vi "单个流程写入.vi"(7 "添加的路径":path, 8 "error in (no error)":errorcluster caption="错误输入（无错误）", 9 "量程":enum16{"低量程", "高量程"}(ring), 10 "测量模式":enum16{"水样测量", "零点核查", "跨度核查", "标样核查", "加标回收"}(ring), 11 "测量参数":enum16{"总磷", "总氮", "氨氮"}(ring)) -> (0 "error out":errorcluster caption="错误输出")   [LabVIEW 2016, in "斯坦道氨氮.lvlib"]
panel:
  out "数组 2":u16[][](array[numeric])
  out "大小":i32
  out "交织的数组":u16[](array[numeric]) format="%04x"
  out "数值":i32
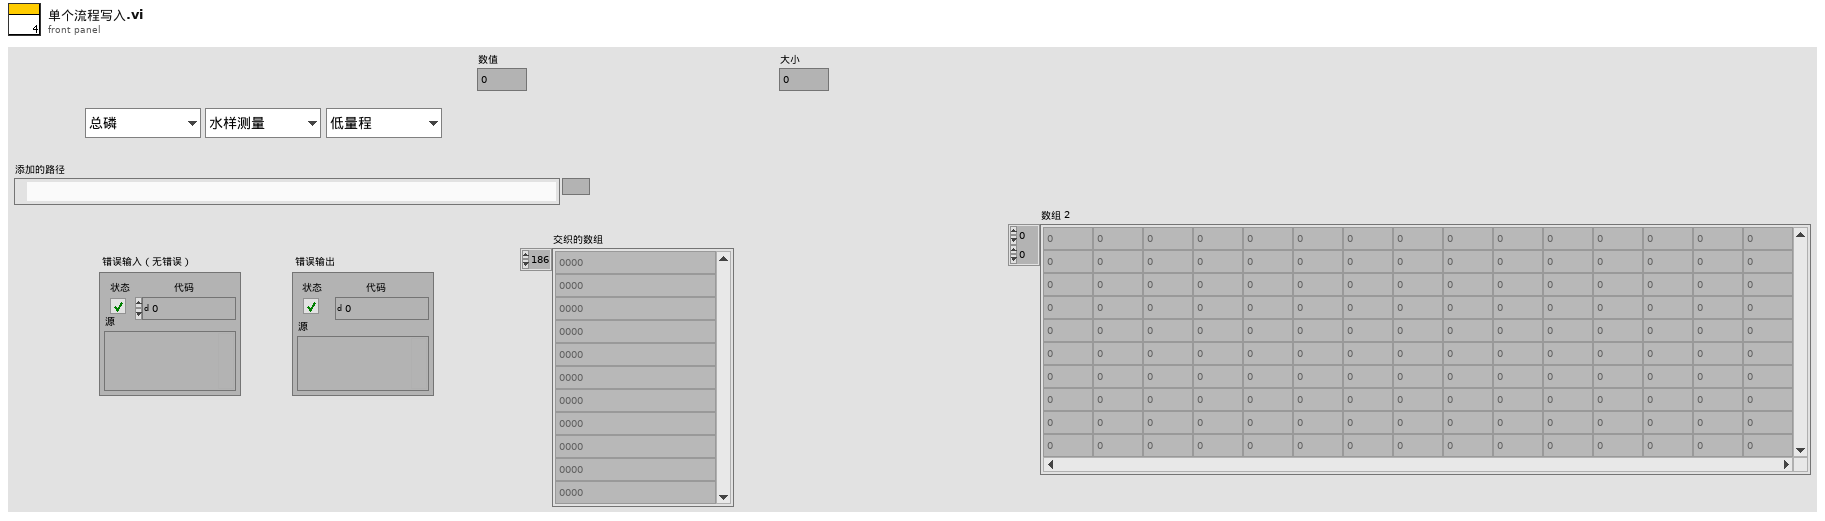
[diagram p1: front panel]
types:
  T1 = cluster{"站号":u16, "starting address":u16, "starting address":u16}
  T2 = cluster{"port":u32, "dac":u8, "adc":u8, "time":u16, "步骤名":string}[]
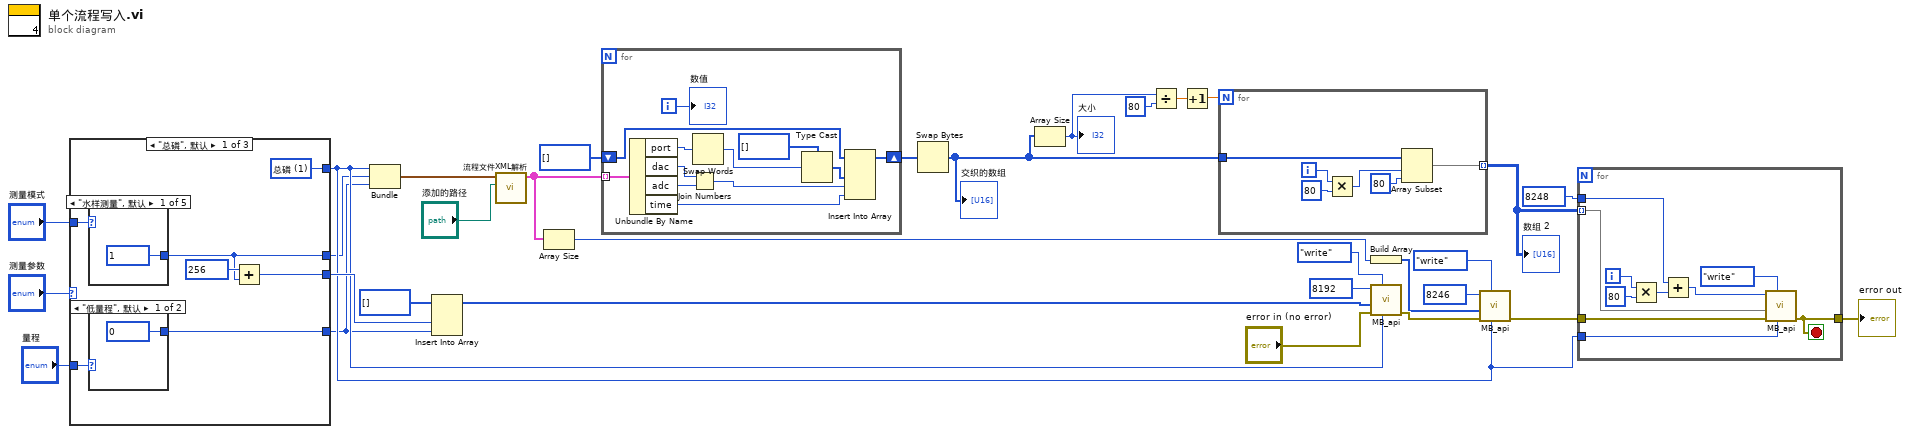
[diagram p0: block diagram]
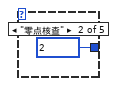
[diagram p2: hidden frame]
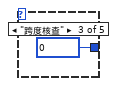
[diagram p3: hidden frame]
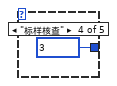
[diagram p4: hidden frame]
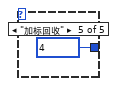
[diagram p5: hidden frame]
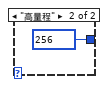
[diagram p6: hidden frame]
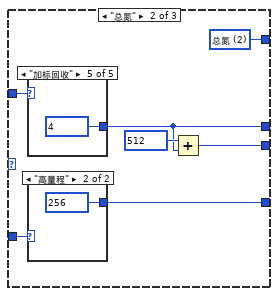
[diagram p7: hidden frame]
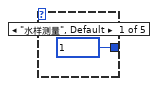
[diagram p8: hidden frame]
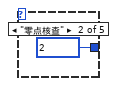
[diagram p9: hidden frame]
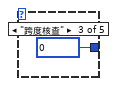
[diagram p10: hidden frame]
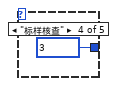
[diagram p11: hidden frame]
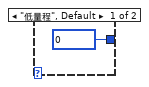
[diagram p12: hidden frame]
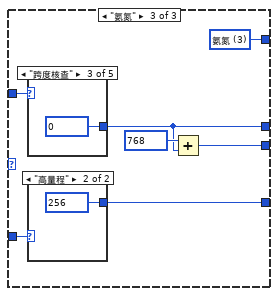
[diagram p13: hidden frame]
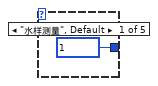
[diagram p14: hidden frame]
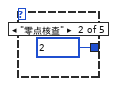
[diagram p15: hidden frame]
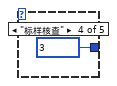
[diagram p16: hidden frame]
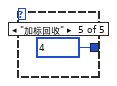
[diagram p17: hidden frame]
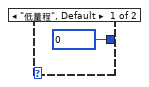
[diagram p18: hidden frame]
diagram:
  n1 = case shown="\"总磷\", 默认" "测量参数" {
    tunnel: "测量模式" -> [w37 w50 w64]
    tunnel: "量程" -> [w38 w51 w65]
    tunnel: [w33 w52 w66] -> w17
    tunnel: [w34 w47 w61] -> w27
    tunnel: [w36 w49 w63] -> w14
    tunnel: [w32 w46 w60] -> w15
    frame "总磷", Default {
      w33 = u16 1 items=["总磷"=1, "总氮"=2, "氨氮"=3] ("站号")
      n2 = case shown="\"水样测量\", 默认" w37 {
        tunnel: [u16 1 ("starting address") u16 2 ("starting address") u16 0 ("starting address") u16 3 ("starting address") u16 4 ("starting address")] -> w32
        frame "水样测量", Default {
        }
        frame "零点核查" {
        }
        frame "跨度核查" {
        }
        frame "标样核查" {
        }
        frame "加标回收" {
        }
      }
      n3 = case shown="\"低量程\", 默认" w38 {
        tunnel: [u16 0 ("starting address") u16 256 ("starting address")] -> w36
        frame "低量程", Default {
        }
        frame "高量程" {
        }
      }
      n4 = Add(x=u16 256 ("starting address"), y=w32) -> (x+y=w34:u16)
    }
    frame "总氮" {
      w52 = u16 2 items=["总磷"=1, "总氮"=2, "氨氮"=3] ("站号")
      n5 = case shown="\"加标回收\"" w50 {
        tunnel: [u16 1 ("starting address") u16 2 ("starting address") u16 0 ("starting address") u16 3 ("starting address") u16 4 ("starting address")] -> w46
        frame "水样测量", Default {
        }
        frame "零点核查" {
        }
        frame "跨度核查" {
        }
        frame "标样核查" {
        }
        frame "加标回收" {
        }
      }
      n6 = case shown="\"高量程\"" w51 {
        tunnel: [u16 0 ("starting address") u16 256 ("starting address")] -> w49
        frame "低量程", Default {
        }
        frame "高量程" {
        }
      }
      n7 = Add(x=u16 512 ("starting address"), y=w46) -> (x+y=w47:u16)
    }
    frame "氨氮" {
      w66 = u16 3 items=["总磷"=1, "总氮"=2, "氨氮"=3] ("站号")
      n8 = case shown="\"跨度核查\"" w64 {
        tunnel: [u16 1 ("starting address") u16 2 ("starting address") u16 0 ("starting address") u16 3 ("starting address") u16 4 ("starting address")] -> w60
        frame "水样测量", Default {
        }
        frame "零点核查" {
        }
        frame "跨度核查" {
        }
        frame "标样核查" {
        }
        frame "加标回收" {
        }
      }
      n9 = case shown="\"高量程\"" w65 {
        tunnel: [u16 0 ("starting address") u16 256 ("starting address")] -> w63
        frame "低量程", Default {
        }
        frame "高量程" {
        }
      }
      n10 = Add(x=u16 768 ("starting address"), y=w60) -> (x+y=w61:u16)
    }
  }
  n11 = Bundle("站号"=w17, "starting address"=w15, "starting address"=w14) -> (w13:T1)  [unwired: 1 in]
  n12 = Insert Into Array(array=u16[] [] ("数组"), new element #1=w27, new element #2=w14) -> (w21:u16[])  [unwired: 1 in]
  n13 = call "流程文件XML解析.vi"("添加的路径"="添加的路径", "参数簇"=w13) -> ("数组"=w5:T2)  [unwired: 9 in]
  n14 = Array Size(array=w5) -> (size(s)=w4:i32)
  n15 = for {
    tunnel: w5 -> [w85] mode=indexing
    shift-right: [w77] -> w10
    shift-left: u16[] [] -> [w75]
    i -> [w84]
    n16 = Unbundle By Name(w85) -> ("port"=w80:u32, "dac"=w83:u8, "adc"=w82:u8, "time"=w78:u16)
    n17 = Join Numbers(hi=w83, lo=w82) -> ((hi.lo)=w79:u16)
    n18 = Swap Words(1:w80) -> (0:w74:u32)
    n19 = Type Cast(type=u16[] [], x=w74) -> (*(type *) &x=w76:u16[])
    n20 = Insert Into Array(array=w75, new element #1=w76, new element #2=w79, new element #3=w78) -> (w77:u16[])  [unwired: 1 in]
    "数值" <- w84
  }
  n21 = Swap Bytes(anything=w10) -> (byte swapped=w7:u16[])
  "交织的数组" <- w7
  n22 = Array Size(array=w7) -> (size(s)=w9:i32)
  "大小" <- w9
  n23 = Divide(x=w9, y=80) -> (x/y=w2:dbl)
  n24 = Increment(x=w2) -> (x+1=w1:dbl)
  n25 = for {
    N: w1 -> [_]
    tunnel: w7 -> [w89]
    tunnel: [w86] -> w6 mode=indexing
    i -> [w91]
    n26 = Multiply(x=w91, y=80) -> (x*y=w88:i32)
    n27 = Array Subset(array=w89, index=w88, length=80 ("y")) -> (w86:u16[])
  }
  "数组 2" <- w6
  n28 = Build Array(w4) -> (w3:i32[])
  n29 = call "MB_api.vi"("Slave ID"=w17, "STEP"=enum16{"open", "read", "write", "close"}."write", "Error in"="error in (no error)", "values"=w21, "starting address"=u16 8192) -> ("error out"=w24:errorcluster)  [unwired: 4 in, 2 out]
  n30 = call "MB_api.vi"("Slave ID"=w17, "STEP"=enum16{"open", "read", "write", "close"}."write", "Error in"=w24, "values"=w3, "starting address"=u16 8246) -> ("error out"=w20:errorcluster)  [unwired: 4 in, 2 out]
  n31 = for {
    tunnel: u16 8248 ("starting address") -> [w95]
    tunnel: w20 -> [w101]
    tunnel: [w99] -> w18
    tunnel: w17 -> [w98]
    tunnel: w6 -> [w97] mode=indexing
    i -> [w94]
    stop <- w99 stop-if-true
    n32 = Multiply(x=w94, y=80) -> (x*y=w93:i32)
    n33 = Add(x=w95, y=w93) -> (x+y=w96:i32)
    n34 = call "MB_api.vi"("Slave ID"=w98, "STEP"=enum16{"open", "read", "write", "close"}."write", "Error in"=w101, "values"=w97, "starting address"=w96) -> ("error out"=w99:errorcluster)  [unwired: 4 in, 2 out]
  }
  "error out" <- w18
